vi "Parallel Executing Test Code.vi"(9 "Test Complete Event":refnum<user-event>, 10 "Positions":u32[](array[numeric]), 11 "MTS Radio Test in":refnum<class "MTS Radio Test.lvclass">) -> ()   [LabVIEW 2015, in "MTS Radio Test.lvclass"]
uses:
  MTS Radio Test.lvclass
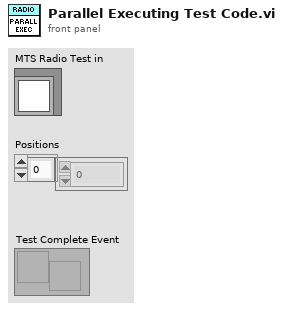
[diagram p1: front panel]
types:
  T1 = cluster{"status":bool, "code":i32, "source":string, "Position":u32}
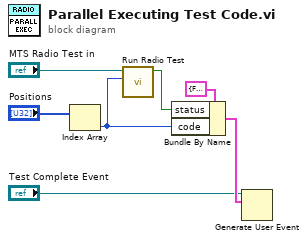
[diagram p0: block diagram]
diagram:
  n1 = Index Array(array="Positions") -> (element=w2:u32)  [unwired: 1 in]
  n2 = call "Run Radio Test.vi"("Position"=w2, "MTS Radio Test in"="MTS Radio Test in") -> ("Passed"=w1:bool)  [unwired: 8 in, 1 out]
  n3 = Bundle By Name(cluster=T1 {"status"=FALSE, "code"=0, "source"="", "Position"=0} ("event data"), "status"=w1, "code"=w2) -> (w7:T1)
  n4 = Generate User Event(user event="Test Complete Event", event data cluster=w7) -> ()  [unwired: 2 in, 2 out]
